vi "mod_PerformResampling.vi"(0 "samples in":cdb[](array[numeric]), 1 "effective filter length":i32, 2 "interpolation factor":i32, 3 "filterData":dbl[](array[numeric]), 5 "resampler state in":T1, 7 "offset":dbl, 9 "rate factor":dbl, 11 "error in (no error)":errorcluster, 12 "reset":bool=TRUE, 13 "flush":bool) -> (4 "samples out":cdb[](array[numeric]), 6 "resampler state out":T1, 15 "error out":errorcluster)   [LabVIEW 2020, in "niAMT.lvlib"]
uses:
  <vilib>/addons/Modulation/niAMT.lvlib
  <vilib>/addons/Modulation/Analog/controls/mod_ResamplerState.ctl
  nilvamt.dll
panel:
  out "return value":i32
  # "This is Ts'/Ts"
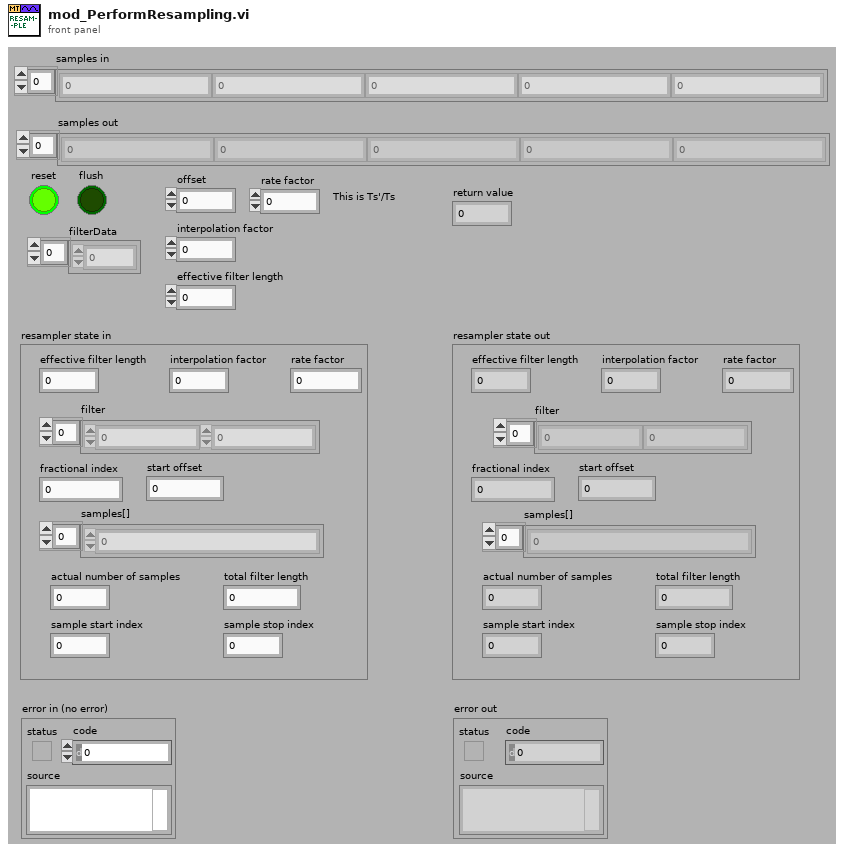
[diagram p1: front panel]
types:
  T1 = typedef "niAMT.lvlib/mod_ResamplerState.ctl" = cluster{"effective filter length":i32, "interpolation factor":i32, "rate factor":dbl, "filter":dbl[], "fractional index":dbl, "start offset":i32, "samples[]":cdb[], "actual number of samples":i32, "total filter length":i32, "sample start index":i32, "sample stop index":i32}
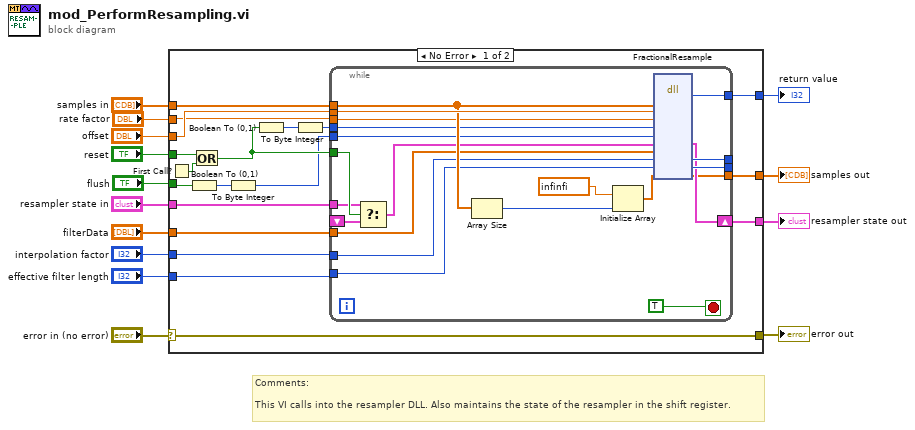
[diagram p0: block diagram]
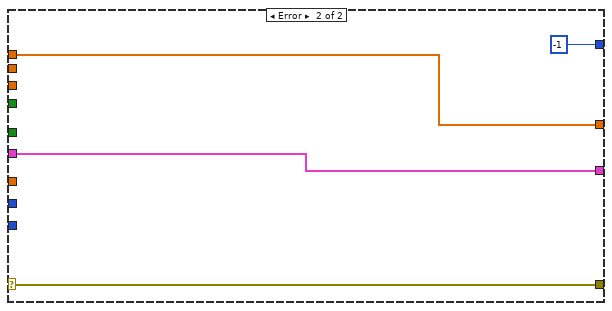
[diagram p2: hidden frame]
diagram:
  # "Comments:\n\nThis VI calls into the resampler DLL. Also maintains the state of the resampler in the shift register."
  n1 = case shown="No Error" "error in (no error)" {
    selector: "error in (no error)" -> [w24 w55]
    tunnel: "samples in" -> [w23 w58]
    tunnel: "resampler state in" -> [w20 w57]
    tunnel: [w33 w57] -> w12
    tunnel: "offset" -> [w32 _]
    tunnel: "reset" -> [w31 _]
    tunnel: "filterData" -> [w28 _]
    tunnel: "interpolation factor" -> [w27 _]
    tunnel: "effective filter length" -> [w26 _]
    tunnel: [w15 w58] -> w6
    tunnel: [w25 -1 ("return type")] -> w5
    tunnel: [w24 w55] -> w3
    tunnel: "rate factor" -> [w19 _]
    tunnel: "flush" -> [w17 _]
    frame No Error {
      n2 = First Call?() -> (First Call?: T/F=w22:bool)
      n3 = Boolean To (0,1)(Boolean=w17) -> (0, 1=w18:i16)
      n4 = Or(x=w31, y=w22) -> (x .or. y?=w21:bool)
      n5 = To Byte Integer(number=w18) -> (8bit integer=w16:i8)
      n6 = Boolean To (0,1)(Boolean=w21) -> (0, 1=w30:i16)
      n7 = To Byte Integer(number=w30) -> (8bit integer=w29:i8)
      n8 = while {
        tunnel: w32 -> [w54]
        tunnel: w29 -> [w44]
        tunnel: w28 -> [w38]
        tunnel: w27 -> [w39]
        tunnel: w26 -> [w40]
        tunnel: [w53] -> _
        tunnel: [w52] -> w25
        tunnel: w23 -> [w49]
        shift-right: [w36] -> w33
        shift-left: _ -> [w46]
        tunnel: w21 -> [w47]
        tunnel: w20 -> [w45]
        tunnel: w19 -> [w43]
        tunnel: [w42] -> _
        tunnel: w16 -> [w35]
        tunnel: [w34] -> w15
        stop <- TRUE stop-if-true
        n9 = Select(t=w45, s=w47, f=w46) -> (s? t:f=w37:T1)
        n10 = Array Size(array=w49) -> (size(s)=w50:i32)
        n11 = Initialize Array(cdb inf+infi ("element"), w50) -> (w41:cdb[])
        n12 = dll-call lib="nilvamt.*" fn="FractionalResample" ("FractionalResampler.dll:FractionalResampleWithNoRateChange")("samples in"=w49, "offset"=w54, "rateFactor"=w43, "reset"=w44, "flush"=w35, "state"=w37, "filterData"=w38, "interpolation factor"=w39, "effective filter length"=w40, "samples out"=w41) -> ("return type"=w52:i32, "state"=w36:T1, "interpolation factor"=w53:i32, "effective filter length"=w42:i32, "samples out"=w34:cdb[])  [unwired: 9 in, 2 out]
      }
    }
    frame Error {
    }
  }
  "samples out" <- w6
  "resampler state out" <- w12
  "return value" <- w5
  "error out" <- w3
